vi "Calibrate Height.vi"(6 "Z Height":dbl, 8 "error in (no error)":errorcluster, 9 "Tip Height":dbl, 10 "XYZTheta In":dbl[](array[numeric]), 11 "Gantry In":refnum<k24>) -> (0 "error out":errorcluster, 3 "Gantry Out":refnum<k24>)   [LabVIEW 2021]
uses:
  C:/Program Files (x86)/Aerotech/A3200/LabVIEW/2010/Bin/Aerotech.A3200.dll
  Program Files (x86)/Aerotech/A3200/LabVIEW/2010/Bin/Aerotech.A3200.dll
  Controller/Motion/Motion.lvclass
  Controller/Motion/A3200/A3200.lvclass
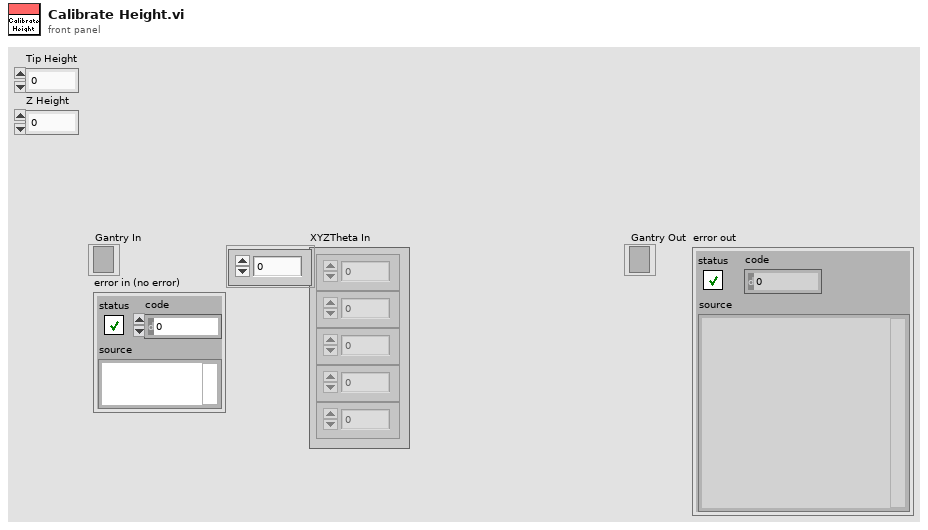
[diagram p1: front panel]
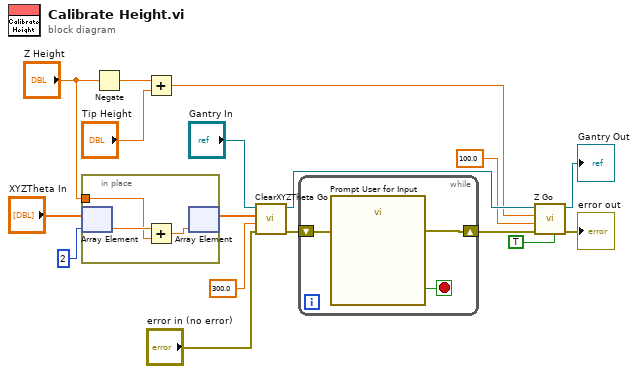
[diagram p0: block diagram]
diagram:
  n1 = in-place {
    in-place-border: "Z Height" -> [w19]
    n2 = in-place-array #1("XYZTheta In", 2) -> (w20:dbl)
    n3 = Add(x=w20, y=w19) -> (x+y=w18:dbl)
    n4 = in-place-array #1(w18) -> (w6:dbl[])  [unwired: 1 out]
  }
  n5 = Negate(x="Z Height") -> (-x=w3:dbl)
  n6 = Add(x=w3, y="Tip Height") -> (x+y=w4:dbl)
  n7 = call "ClearXYZTheta Go.vi"("error in (no error)"="error in (no error)", "Speed"=300.0, "XYZTheta In"=w6, "Gantry In"="Gantry In") -> ("error out"=w14:errorcluster, "Gantry Out"=w13:refnum<k24>)  [unwired: 5 in, 1 out]
  n8 = while {
    shift-right: [w21] -> w10
    shift-left: w14 -> [w22]
    stop <- w23 stop-if-true
    n9 = call "Prompt User for Input"("error in (no error)"=w22) -> ("Tip on component?"=w23:bool, "error out"=w21:errorcluster)  [unwired: 16 in, 1 out]
  }
  n10 = call "Z Go.vi"("Increment"=TRUE, "error in (no error)"=w10, "Speed In"=100.0, "Position In"=w4, "Gantry In"=w13) -> ("error out"=→"error out":errorcluster, "Gantry Out"=→"Gantry Out":refnum<k24>)  [unwired: 3 in, 2 out]
